vi "PublishMqtt.vi"(9 "Light":dbl, 10 "pH":dbl, 11 "Temp":dbl) -> (3 "Publisher Message":string)   [LabVIEW 2022 SP3]
panel:
  in  "Python path":path
  out "Subscriber Message":string
  in  "module path":path
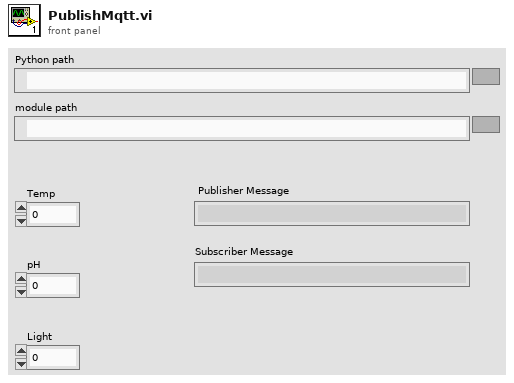
[diagram p1: front panel]
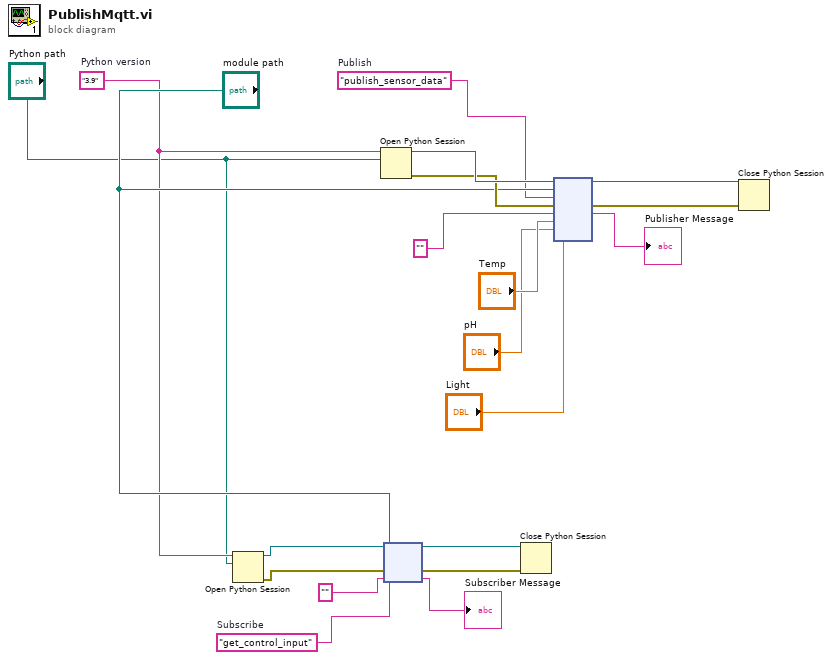
[diagram p0: block diagram]
diagram:
  w1 = "get_control_input"  # Subscribe
  w2 = "publish_sensor_data"  # Publish
  w4 = "3.9"  # Python version
  n1 = Open Python Session(python version=w4, python path="Python path") -> (session out=w12:refnum<k35>, error out=w11:errorcluster)  [unwired: 1 in]
  n2 = Open Python Session(python version=w4, python path="Python path") -> (session out=w20:refnum<k35>, error out=w15:errorcluster)  [unwired: 1 in]
  n3 = node(w12, "module path", w1, w11, "") -> (w10:refnum<k35>, w9:errorcluster, →"Subscriber Message":string)  [unwired: 2 out]
  n4 = Close Python Session(session in=w10, error in=w9) -> ()  [unwired: 1 out]
  n5 = node(w20, "module path", w2, w15, "", "Temp", "pH", "Light") -> (w19:refnum<k35>, w14:errorcluster, →"Publisher Message":string)  [unwired: 3 in, 2 out]
  n6 = Close Python Session(session in=w19, error in=w14) -> ()  [unwired: 1 out]
